vi "split object path to hierarchy local.vi"(11 "Object path":string="IndivITX/Test1/SA03008N.20190801.000000.itx") -> (1 "parent path":string, 2 "layers":i32, 3 "hierarchy":string[](array[string]))   [LabVIEW 2016]
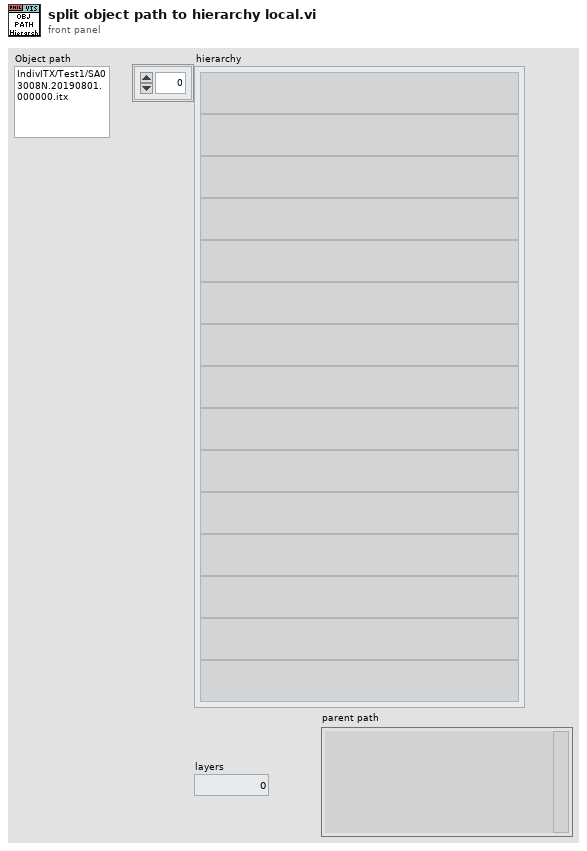
[diagram p1: front panel]
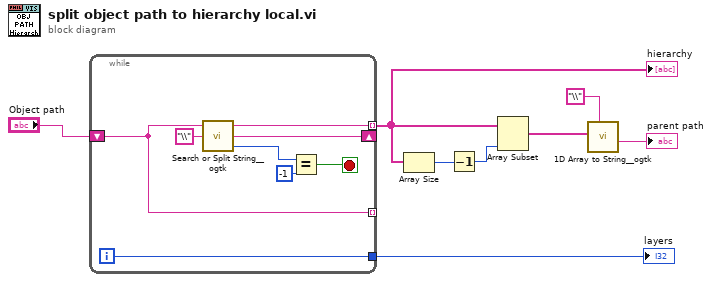
[diagram p0: block diagram]
diagram:
  n1 = while {
    shift-right: [w12] -> _
    shift-left: "Object path" -> [w13]
    tunnel: [w13] -> _ mode=indexing
    tunnel: [w11] -> w7
    tunnel: [w10] -> w2 mode=indexing
    i -> [w11]
    stop <- w14 stop-if-true
    n2 = call <userlib>:"Search or Split String__ogtk.vi"("search string/char (-)"="\\", "string"=w13) -> ("offset after match"=w9:i32, "substring after match"=w12:string, "substring before match"=w10:string)  [unwired: 1 in]
    n3 = Equal?(x=w9, y=-1) -> (x = y?=w14:bool)
  }
  "hierarchy" <- w2
  "layers" <- w7
  n4 = Array Size(array=w2) -> (size(s)=w6:i32)
  n5 = Decrement(x=w6) -> (x-1=w1:i32)
  n6 = Array Subset(array=w2, length=w1) -> (w5:string[])  [unwired: 1 in]
  n7 = call <userlib>:"1D Array to String__ogtk.vi"("delimiter (Tab)"="\\", "Array of Strings"=w5) -> ("delimited string"=→"parent path":string)  [unwired: 9 in]
